vi "Find and export an FPGA Addon Configuration.vi"() -> ()   [LabVIEW 2020]
uses:
  <vilib>/addons/VeriStand Custom Device Scripting APIs/FPGA Addon/Scripting API.lvlibp
panel:
  out "Exported location":path
  out "error out":errorcluster
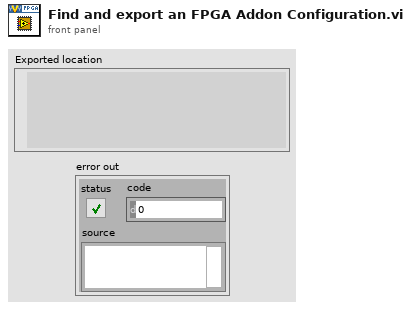
[diagram p1: front panel]
types:
  T1 = typedef "Scripting API.lvlibp/Custom Device API.lvlib/Custom Device Item Ref.ctl" = u64
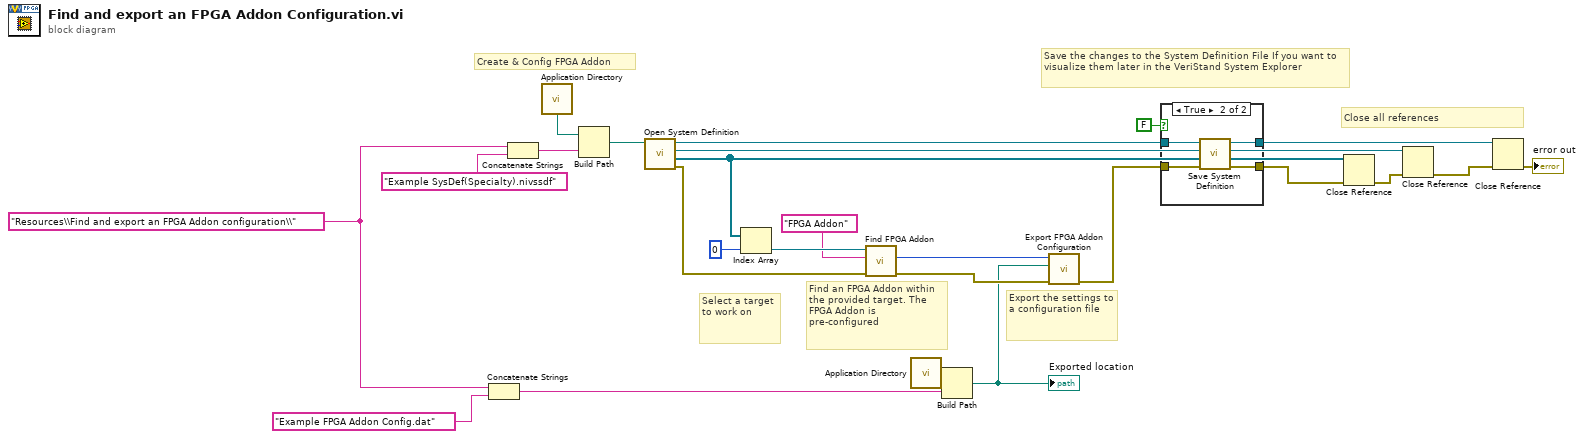
[diagram p0: block diagram]
diagram:
  w11 = "Resources\\Find and export an FPGA Addon configuration\\" ("name or relative path")
  # "Create & Config FPGA Addon"
  # "Export the settings to a configuration file"
  # "Save the changes to the System Definition File If you want to visualize them later in the VeriStand System Explorer"
  # "Close all references"
  # "Find an FPGA Addon within the provided target. The FPGA Addon is pre-configured"
  # "Select a target to work on"
  n1 = Concatenate Strings(w11, "Example FPGA Addon Config.dat" ("name or relative path")) -> (w9:string)
  n2 = Concatenate Strings(w11, "Example SysDef(Specialty).nivssdf" ("name or relative path")) -> (w12:string)
  n3 = call <vilib>:"Application Directory.vi"() -> ("Application Directory"=w20:path)
  n4 = Build Path(base path=w20, name or relative path=w12) -> (appended path=w19:path)
  n5 = call "Open System Definition.vi"("System Definition File"=w19) -> ("error out"=w4:errorcluster, "targets refnums"=w23:refnum<k24>[], "root refnum"=w24:refnum<k24>, "system definition refnum"=w17:refnum<k24>)  [unwired: 7 in]
  n6 = Index Array(array=w23, index=0) -> (element=w7:refnum<k24>)
  n7 = call <vilib>:"Find FPGA Addon.vi"("error in"=w4, "FPGA addon name"="FPGA Addon" ("fpga addon name"), "target in"=w7) -> ("error out"=w5:errorcluster, "FPGA addon refnum out"=w3:T1)  [unwired: 5 in, 2 out]
  n8 = call <vilib>:"Application Directory.vi"() -> ("Application Directory"=w14:path)
  n9 = Build Path(base path=w14, name or relative path=w9) -> (appended path=w2:path)
  "Exported location" <- w2
  n10 = call <vilib>:"Export FPGA Addon Configuration.vi"("error in"=w5, "export file path"=w2, "FPGA addon refnum in"=w3) -> ("error out"=w1:errorcluster)  [unwired: 7 in, 1 out]
  n11 = case shown="True" FALSE {
    tunnel: w17 -> [w27 w31]
    tunnel: [w27 w30] -> w16
    tunnel: [w26 w29] -> w15
    tunnel: w1 -> [w26 w28]
    frame False {
    }
    frame True {
      n12 = call "Save System Definition.vi"("error in (no error)"=w28, ".NET Refnum in"=w31) -> ("error out"=w29:errorcluster, ".NET Refnum out"=w30:refnum<k24>)  [unwired: 8 in]
    }
  }
  n13 = Close Reference(reference=w23, error in (no error)=w15) -> (error out=w22:errorcluster)
  n14 = Close Reference(reference=w24, error in (no error)=w22) -> (error out=w21:errorcluster)
  n15 = Close Reference(reference=w16, error in (no error)=w21) -> (error out=→"error out":errorcluster)
